vi "Installation.vi"() -> ()   [LabVIEW 2020]
uses:
  <vilib>/registry/registry.llb/Registry RtKey.ctl
  <vilib>/registry/registry.llb/Read Registry Value Simple STR.vi
  <vilib>/registry/registry.llb/Write Registry Value Simple STR.vi
  <vilib>/regexp/Match Regular Expression.xnode
panel:
  out "curl command":string
  out "Error install sklearn":errorcluster
  out "Error Write Environment Variable":errorcluster
  out "Error Python installation":errorcluster
  out "Windows?":bool
  out "Python installation":string
  out "Error Read Environment Variable":errorcluster
  out "String/Binary data":string
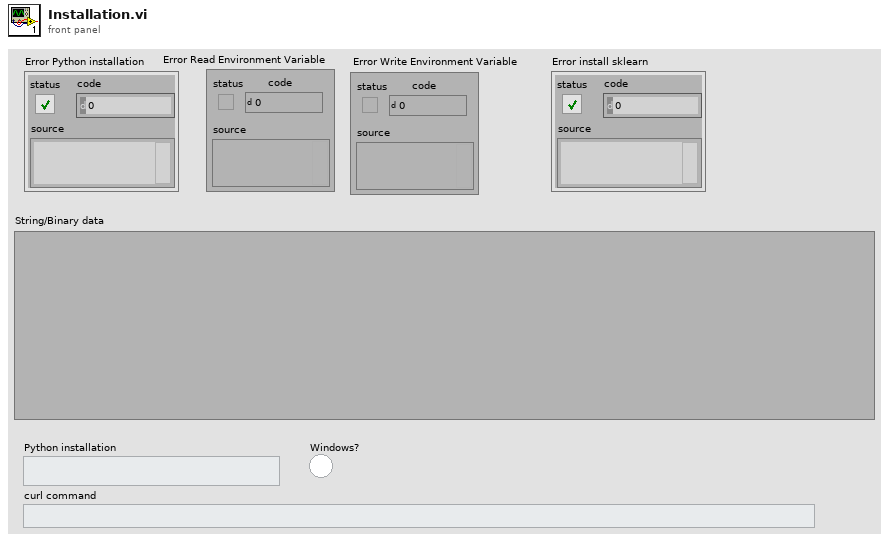
[diagram p1: front panel]
types:
  T1 = typedef "Registry RtKey.ctl" = enum32{"HKEY_CLASSES_ROOT", "HKEY_CURRENT_USER", "HKEY_LOCAL_MACHINE", "HKEY_USERS", "HKEY_PERFORMANCE_DATA", "HKEY_CURRENT_CONFIG", "HKEY_DYN_DATA"}
  T2 = typedef "Registry refnum.ctl" = refnum<k1>
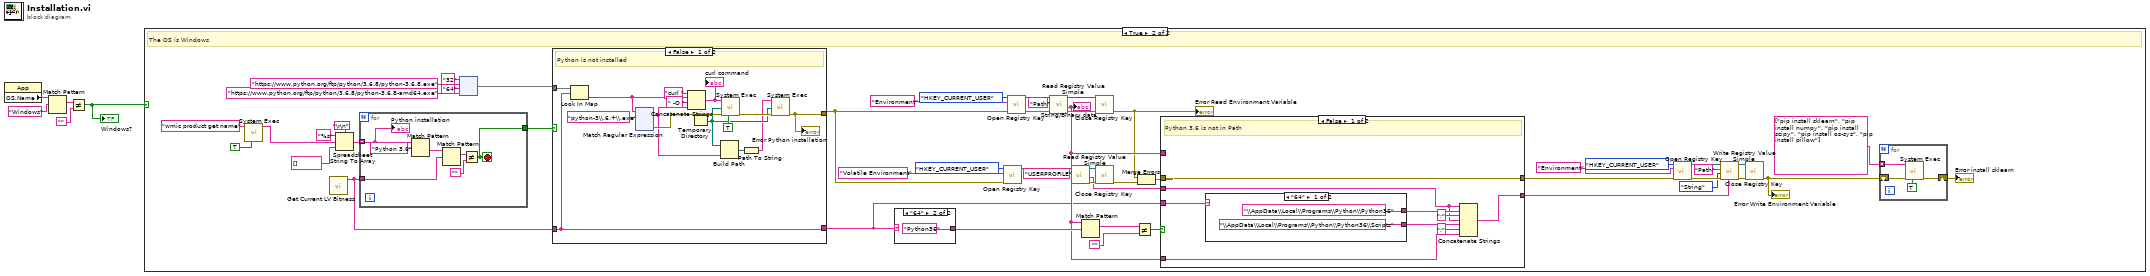
[diagram p0: block diagram]
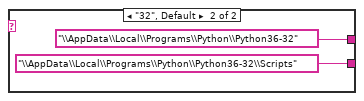
[diagram p4: hidden frame]
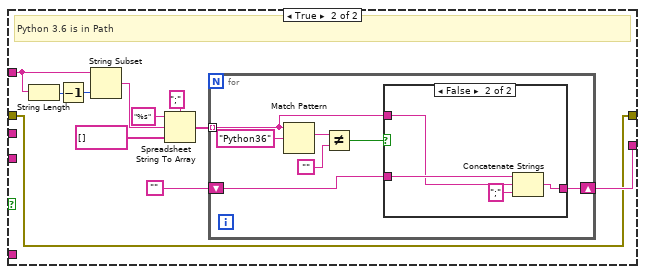
[diagram p5: hidden frame]
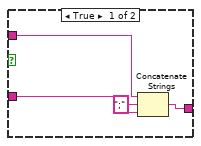
[diagram p6: hidden frame]
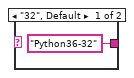
[diagram p7: hidden frame]
diagram:
  n1 = property class="App"() -> ("OS.Name"=w5:string)  [unwired: 2 in, 2 out]
  n2 = Match Pattern(string=w5, regular expression="Windows") -> (match substring=w3:string)  [unwired: 1 in, 3 out]
  n3 = Not Equal?(x=w3, y="") -> (x != y?=w1:bool)
  "Windows?" <- w1
  n4 = case shown="True" w1 {
    frame False {
    }
    frame True {
      # "The OS is Windows"
      n5 = call <vilib>:"System Exec.vi"("run minimized? (F)"=TRUE, "command line"="wmic product get name") -> ("standard output"=w55:string)  [unwired: 6 in, 3 out]
      n6 = call <vilib>:"Get Current LV Bitness.vi"() -> ("bitness"=w43:string)  [unwired: 11 in]
      n7 = Spreadsheet String To Array(delimiter (Tab)="\r\n", format string="%s", spreadsheet string=w55, array type (2D Dbl)=string[] []) -> (array=w51:string[])
      n8 = for {
        tunnel: w51 -> [w197] mode=indexing
        tunnel: w43 -> [w195]
        tunnel: [w191] -> w49
        stop <- w191 stop-if-true
        n9 = Match Pattern(string=w197, regular expression="Python 3.6") -> (after substring=w192:string)  [unwired: 1 in, 3 out]
        n10 = Match Pattern(string=w192, regular expression=w195) -> (match substring=w194:string)  [unwired: 1 in, 3 out]
        n11 = Not Equal?(x=w194, y="") -> (x != y?=w191:bool)
        "Python installation" <- w197
      }
      n12 = node("32" ("key"), "https://www.python.org/ftp/python/3.6.8/python-3.6.8.exe", "64" ("key"), "https://www.python.org/ftp/python/3.6.8/python-3.6.8-amd64.exe") -> (w44:map{string, string})
      n13 = case shown="False" w49 {
        tunnel: w44 -> [w75 _]
        tunnel: w43 -> [w66 w190]
        tunnel: [w67 _] -> w12
        tunnel: [w66 w190] -> w7
        frame False {
          # "Python is not installed"
          n14 = Look In Map(map=w75, key=w66) -> (value=w70:string)  [unwired: 1 in, 1 out]
          n15 = xnode "Match Regular Expression"("input string"=w70, "regular expression"="python-3\\.6.+\\.exe") -> ("whole match"=w62:string, "error out"=w68:errorcluster)  [unwired: 4 in, 3 out]
          n16 = Concatenate Strings("curl " ("string"), w70, " -O " ("string"), w62) -> (w73:string)
          "curl command" <- w73
          n17 = Temporary Directory() -> (w63:path)
          n18 = Build Path(base path=w63, name or relative path=w62) -> (appended path=w64:path)
          n19 = call <vilib>:"System Exec.vi"("run minimized? (F)"=TRUE ("wait until completion? (T)"), "error in (no error)"=w68, "working directory"=w63, "command line"=w73) -> ("error out"=w72:errorcluster)  [unwired: 4 in, 3 out]
          n20 = Path To String(path=w64) -> (string=w61:string)
          n21 = call <vilib>:"System Exec.vi"("error in (no error)"=w72, "working directory"=w63, "command line"=w61) -> ("error out"=w67:errorcluster)  [unwired: 5 in, 3 out]
          "Error Python installation" <- w67
        }
        frame True {
          # "Python is installed"
        }
      }
      n22 = case shown="\"64\"" w7 {
        tunnel: ["Python36-32" "Python36"] -> w35
        frame "32", Default {
        }
        frame "64" {
        }
      }
      n23 = call <vilib>:"Open Registry Key.vi"("error in (no error)"=w12, "subkey"="Volatile Environment", "root key (HKEY_LOCAL_MACHINE)"=Registry_RtKey."HKEY_CURRENT_USER") -> ("refnum out"=w17:T2)  [unwired: 7 in, 1 out]
      n24 = call <vilib>:"Open Registry Key.vi"("error in (no error)"=w12, "subkey"="Environment", "root key (HKEY_LOCAL_MACHINE)"=Registry_RtKey."HKEY_CURRENT_USER") -> ("error out"=w37:errorcluster, "refnum out"=w40:T2)  [unwired: 7 in]
      n25 = call-poly <vilib>:"Read Registry Value Simple.vi"("error in (no error)"=w37, "value"="Path", "refnum"=w40) -> ("error out"=w36:errorcluster, "String/Binary data"=w31:string, "refnum out"=w38:T2)  [unwired: 3 in, 1 out]
      "String/Binary data" <- w31
      n26 = call-poly <vilib>:"Read Registry Value Simple.vi"("value"="USERPROFILE", "refnum"=w17) -> ("error out"=w14:errorcluster, "String/Binary data"=w11:string, "refnum out"=w16:T2)  [unwired: 4 in, 1 out]
      n27 = Match Pattern(string=w31, regular expression=w35) -> (match substring=w34:string)  [unwired: 1 in, 3 out]
      n28 = call <vilib>:"Close Registry Key.vi"("error in (no error)"=w36, "refnum"=w38) -> ("error out"=w9:errorcluster)  [unwired: 5 in]
      "Error Read Environment Variable" <- w9
      n29 = call <vilib>:"Close Registry Key.vi"("error in (no error)"=w14, "refnum"=w16) -> ("error out"=w8:errorcluster)  [unwired: 5 in]
      n30 = Not Equal?(x=w34, y="") -> (x != y?=w32:bool)
      n31 = Merge Errors(w9, w8) -> (w10:errorcluster)
      n32 = case shown="False" w32 {
        tunnel: w10 -> [w206 w211]
        tunnel: w31 -> [_ w216]
        tunnel: w31 -> [w201 _]
        tunnel: [w206 w211] -> w26
        tunnel: [w200 w212] -> w23
        tunnel: w11 -> [w199 _]
        tunnel: w7 -> [w198 _]
        frame False {
          # "Python 3.6 is not in Path"
          n33 = case shown="\"64\"" w198 {
            tunnel: ["\\AppData\\Local\\Programs\\Python\\Python36" ("string") "\\AppData\\Local\\Programs\\Python\\Python36-32" ("string")] -> w205
            tunnel: ["\\AppData\\Local\\Programs\\Python\\Python36\\Scripts" ("string") "\\AppData\\Local\\Programs\\Python\\Python36-32\\Scripts" ("string")] -> w203
            frame "64" {
            }
            frame "32", Default {
            }
          }
          n34 = Concatenate Strings(w199, w205, ";" ("string"), w199, w203, ";" ("string"), w201) -> (w200:string)
        }
        frame True {
          # "Python 3.6 is in Path"
          n35 = String Length(string=w216) -> (length=w215:i32)
          n36 = Decrement(x=w215) -> (x-1=w214:i32)
          n37 = String Subset(string=w216, length (rest)=w214) -> (substring=w213:string)  [unwired: 1 in]
          n38 = Spreadsheet String To Array(delimiter (Tab)=";", format string="%s", spreadsheet string=w213, array type (2D Dbl)=string[] []) -> (array=w218:string[])
          n39 = for {
            tunnel: w218 -> [w224] mode=indexing
            shift-right: [w222] -> w212
            shift-left: "" -> [w223]
            n40 = Match Pattern(string=w224, regular expression="Python36") -> (match substring=w227:string)  [unwired: 1 in, 3 out]
            n41 = Not Equal?(x=w227, y="") -> (x != y?=w225:bool)
            n42 = case shown="False" w225 {
              tunnel: w224 -> [w232 w234]
              tunnel: w223 -> [w229 w236]
              tunnel: [w231 w235] -> w222
              frame True {
                n43 = Concatenate Strings(w232, ";" ("string"), w229) -> (w231:string)
              }
              frame False {
                n44 = Concatenate Strings(w236, w234, ";" ("string")) -> (w235:string)
              }
            }
          }
        }
      }
      n45 = call <vilib>:"Open Registry Key.vi"("error in (no error)"=w26, "subkey"="Environment", "root key (HKEY_LOCAL_MACHINE)"=Registry_RtKey."HKEY_CURRENT_USER") -> ("error out"=w29:errorcluster, "refnum out"=w27:T2)  [unwired: 7 in]
      n46 = call-poly <vilib>:"Write Registry Value Simple.vi"("String/Binary data"=w23, "error in (no error)"=w29, "simple data type"=enum16{"String", "Binary", "DWORD"}."String", "value"="Path", "refnum"=w27) -> ("error out"=w30:errorcluster, "refnum out"=w28:T2)  [unwired: 3 in]
      n47 = call <vilib>:"Close Registry Key.vi"("error in (no error)"=w30, "refnum"=w28) -> ("error out"=w20:errorcluster)  [unwired: 5 in]
      "Error Write Environment Variable" <- w20
      n48 = for {
        shift-right: [w59] -> w19
        shift-left: w20 -> [w60]
        tunnel: string[] ["pip install sklearn", "pip install numpy", "pip install scipy", "pip install os-sys", "pip install pillow"] -> [w57] mode=indexing
        n49 = call <vilib>:"System Exec.vi"("run minimized? (F)"=TRUE, "error in (no error)"=w60, "command line"=w57) -> ("error out"=w59:errorcluster)  [unwired: 5 in, 3 out]
      }
      "Error install sklearn" <- w19
    }
  }
